vi "Write CAN.IoMode.vi"(8 "error in (no error)":errorcluster, 10 "CAN.IoMode":u32, 11 "database file in":refnum<class "database file.lvclass">) -> (0 "error out":errorcluster, 3 "database file out":refnum<class "database file.lvclass">)   [LabVIEW 2013, in "database file.lvclass"]
uses:
  database file.lvclass
  database file.lvclass/database file.ctl
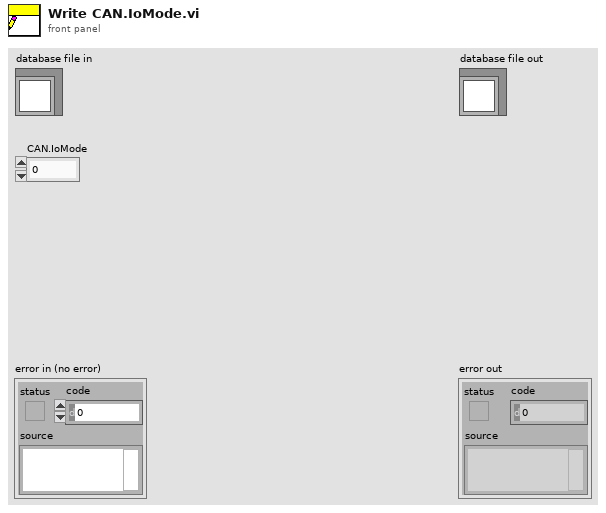
[diagram p1: front panel]
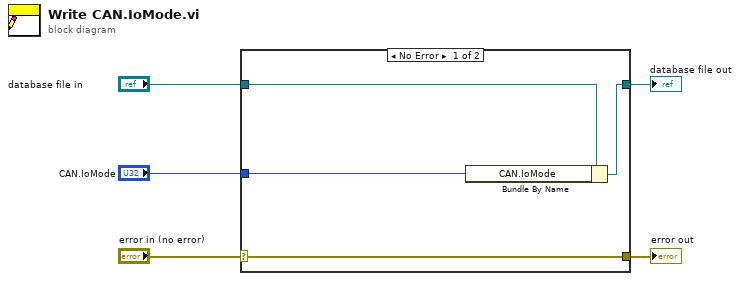
[diagram p0: block diagram]
diagram:
  n1 = case shown="No Error" "error in (no error)" {
    selector: "error in (no error)" -> [w9 w10]
    tunnel: [w9 w10] -> w4
    tunnel: [w7 w11] -> w2
    tunnel: "database file in" -> [w8 w11]
    tunnel: "CAN.IoMode" -> [w6 _]
    frame No Error {
      n2 = Bundle By Name(cluster=w8, "CAN.IoMode"=w6) -> (w7:refnum<class "database file.lvclass">)
    }
    frame Error {
    }
  }
  "error out" <- w4
  "database file out" <- w2
